vi "writes_data.vi"(0 "Path":path, 5 "Key":string, 9 "Value":dbl, 11 "error in (no error)":errorcluster) -> (15 "error out":errorcluster)   [LabVIEW 2023]
uses:
  <vilib>/Utility/config.llb/Write Key (Double).vi
  <vilib>/Utility/config.llb/NI_LVConfig.lvlib
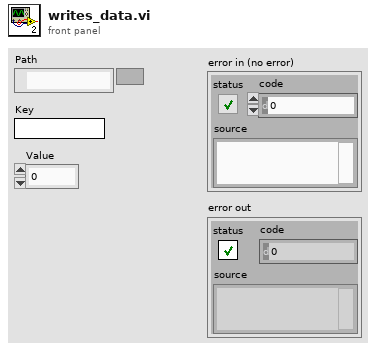
[diagram p1: front panel]
types:
  T1 = typedef "NI_LVConfig.lvlib/Config Data RefNum.ctl" = refnum<k1>
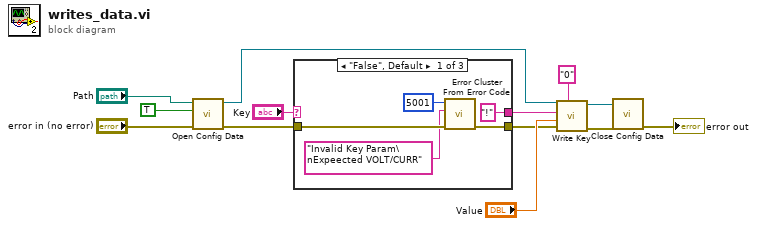
[diagram p0: block diagram]
diagram:
  n1 = call <vilib>:"Open Config Data.vi"("error in (no error)"="error in (no error)", "create file if necessary (T)"=TRUE, "configuration file path"="Path") -> ("error out"=w2:errorcluster, "refnum"=w7:T1)  [unwired: 6 in, 1 out]
  n2 = case shown="\"False\", Default" "Key" {
    selector: "Key" -> [_ w20 w22]
    tunnel: ["!" w20 w22] -> w3
    tunnel: w2 -> [w18 w19 w21]
    tunnel: [w16 w19 w21] -> w1
    frame "False", Default {
      n3 = call <vilib>:"Error Cluster From Error Code.vi"("error in (no error)"=w18, "error message (\"\")"="Invalid Key Param\nExpeected VOLT/CURR" ("error message (\"\")"), "error code (0)"=5001) -> ("error out"=w16:errorcluster)  [unwired: 6 in]
    }
    frame "CURR" {
    }
    frame "VOLT" {
    }
  }
  n4 = call-poly <vilib>:"Write Key.vi"("section"="0", "error in (no error)"=w1, "value"="Value", "key"=w3, "refnum"=w7) -> ("error out"=w5:errorcluster, "refnum out"=w9:T1)  [unwired: 4 in, 1 out]
  n5 = call <vilib>:"Close Config Data.vi"("error in (no error)"=w5, "refnum"=w9) -> ("error out"=→"error out":errorcluster)  [unwired: 8 in, 1 out]
